vi "Save File.vi"(8 "error in (no error)":errorcluster, 9 "Data (\"\")":string, 10 "Operation (0 : Open)":T1(ring), 11 "File Path (\"\")":path) -> (0 "error out":errorcluster)   [LabVIEW 2020, in "Yokogawa GX Series.lvlib"]
doc: "This VI converts Measurement Binary Data to array of Blocks."
uses:
  <instrlib>/Yokogawa GX Series/Yokogawa GX Series.lvlib
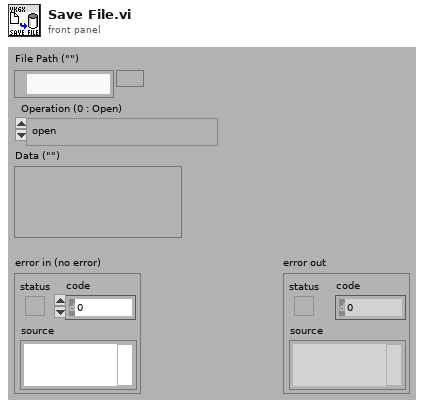
[diagram p1: front panel]
types:
  T1 = enum16{"open", "replace", "create", "open or create", "replace or create", "replace or create with confirmation"}
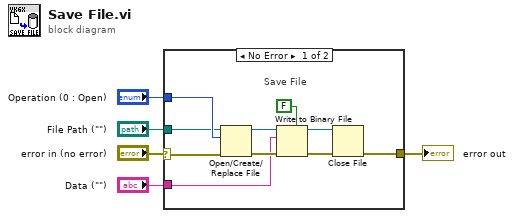
[diagram p0: block diagram]
diagram:
  n1 = case shown="No Error" "error in (no error)" {
    selector: "error in (no error)" -> [w6 w16]
    tunnel: [w10 w16] -> w5
    tunnel: "Data (\"\")" -> [w9 _]
    tunnel: "Operation (0 : Open)" -> [w8 _]
    tunnel: "File Path (\"\")" -> [w7 _]
    frame No Error {
      # "Save File"
      n2 = Open/Create/Replace File(file path (use dialog)=w7, error in=w6, operation (0:open)=w8) -> (refnum out=w13:refnum<file>, error out=w11:errorcluster)  [unwired: 3 in, 1 out]
      n3 = Write to Binary File(file (use dialog)=w13, data=w9, error in=w11, 5:FALSE ("配列または文字列サイズを先頭に追加?(T)")) -> (refnum out=w14:refnum<file>, error out=w12:errorcluster)  [unwired: 3 out]
      n4 = Close File(refnum=w14, error in=w12) -> (error out=w10:errorcluster)  [unwired: 1 out]
    }
    frame Error {
    }
  }
  "error out" <- w5
